vi "WriteL.vi"(0 "val":u32, 1 "board":u32, 2 "offset":u32) -> ()   [LabVIEW 2015]
uses:
  lv64_eventdriven2015/board.vis/ESLSCDLL.dll
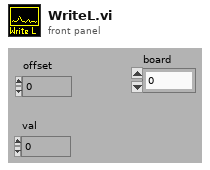
[diagram p1: front panel]
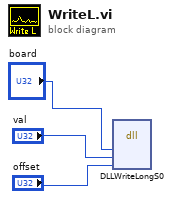
[diagram p0: block diagram]
diagram:
  n1 = dll-call lib="C:/ENTW/PCIE/64bit/lv64/lv64_eventdriven2015/board.vis/ESLSCDLL.dll" fn="DLLWriteLongS0"("drv"="board", "DataByte"="val", "PortOff"="offset") -> ()  [unwired: 7 in, 2 out]
